vi "Constructor by Table.vi"(8 "error in (no error)":errorcluster, 9 "Field Factory Type":refnum<class "Column Factory.lvclass">, 10 "Configured Table":refnum<class "Basic Table.lvclass">, 11 "Form from Configured Table in":refnum<class "Form from Configured Table.lvclass">) -> (0 "error out":errorcluster, 3 "Form from Configured Table out":refnum<class "Form from Configured Table.lvclass">)   [LabVIEW 2020, in "Panel Form Controller.lvlib" / "Form from Configured Table.lvclass"]
uses:
  Form from Configured Table.lvclass
  C:/Users/User/Desktop/Raman Program/Database OOP/source/Forms AF/Forms Controller/Configuration/Controller Configuration/Panel Form Controller Configuration.lvclass
  Database OOP/Table Libraries/Basic Table/Basic Table Class/Basic Table.lvclass
  Database OOP/Column Libraries/Basic Columns/Column Configuration/Column Factory Parent Class/Column Factory.lvclass
  Form from Configured Table.lvclass/Form from Configured Table.ctl
  Controller Configuration/Panel Form Controller Configuration.lvclass/Panel Form Controller Configuration.ctl
  Controller Configuration/Panel Form Controller Configuration.lvclass
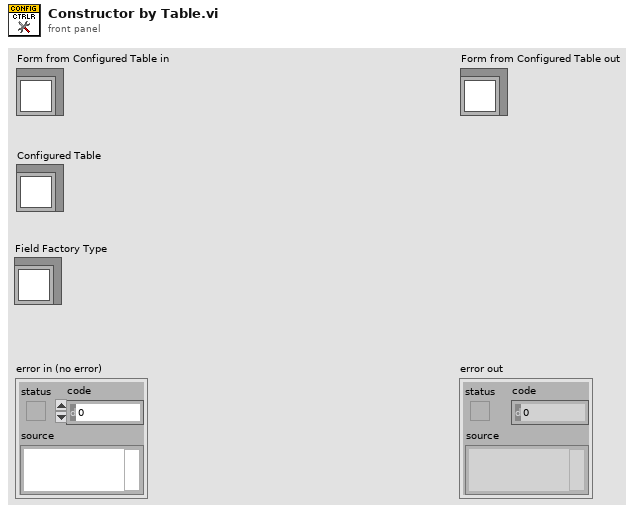
[diagram p1: front panel]
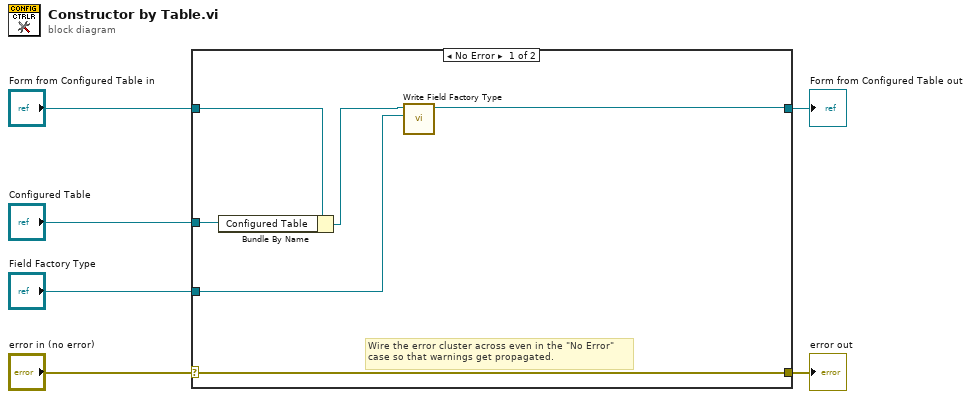
[diagram p0: block diagram]
diagram:
  n1 = case shown="No Error" "error in (no error)" {
    selector: "error in (no error)" -> [w12 w14]
    tunnel: [w12 w14] -> w5
    tunnel: [w7 w13] -> w3
    tunnel: "Form from Configured Table in" -> [w11 w13]
    tunnel: "Configured Table" -> [w10 _]
    tunnel: "Field Factory Type" -> [w9 _]
    frame No Error {
      # "Wire the error cluster across even in the \"No Error\"\ncase so that warnings get propagated."
      n2 = Bundle By Name(cluster=w11, "Configured Table"=w10) -> (w8:refnum<class "Form from Configured Table.lvclass">)
      n3 = call "Write Field Factory Type.vi"("Field Factory Type"=w9, "Panel Form Controller Configuration in"=w8) -> ("Panel Form Controller Configuration out"=w7:refnum<class "Form from Configured Table.lvclass">)  [unwired: 8 in, 1 out]
    }
    frame Error {
    }
  }
  "error out" <- w5
  "Form from Configured Table out" <- w3
